vi "Receive Value Change Event.vi"(8 "error in (no error)":errorcluster, 10 "ValueChangeMsg":refnum<class "ValueChangeMsg.lvclass">, 11 "PauseResumeButtons In":refnum<class "PauseResumeButtons.lvclass">) -> (0 "error out":errorcluster, 3 "PauseResumeButtons Out":refnum<class "PauseResumeButtons.lvclass">)   [LabVIEW 2020, in "MVAExamples.lvlib" / "PauseResumeButtons.lvclass"]
doc: "<License>\nCopyright © 2017 Composed Systems, LLC | All rights reserved\nwww.composed.io\n\nAuthor: Ethan Stern <ethan.stern@composed.io>\n\nThis software is provided \"AS IS\" WITHOUT WARRANTIES, either express or implied, AND IS FOR EDUCATIONAL PURPOSES ONLY.\n</License>"
uses:
  PauseResumeButtons.lvclass
  modules/mva-viewable/Source/ActorEvents/IEventAggregator Messages/ValueChangeMsg/ValueChangeMsg.lvclass
  modules/mva-viewable/Source/ActorEvents/IEventAggregator Messages/ValueChangeMsg/ValueChangeMsg.lvclass/ValueChangeMsg.ctl
  PauseResumeButtons.lvclass/PauseResumeButtons.ctl
  modules/mva-viewable/Source/ActorEvents/IEventAggregator Messages/ValueChangeMsg/Accessors/Read Control Label.vi
  modules/mva-viewable/Source/IViewable/IViewable/IViewable.lvclass
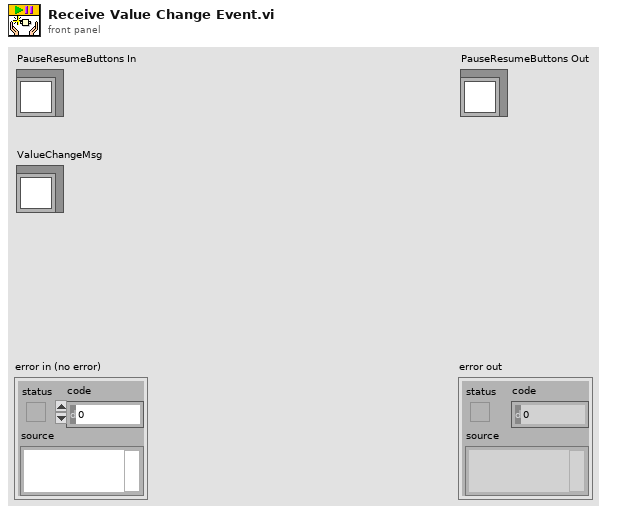
[diagram p1: front panel]
types:
  T1 = enum8{"Enabled", "Disabled", "Disabled and Grayed Out"}
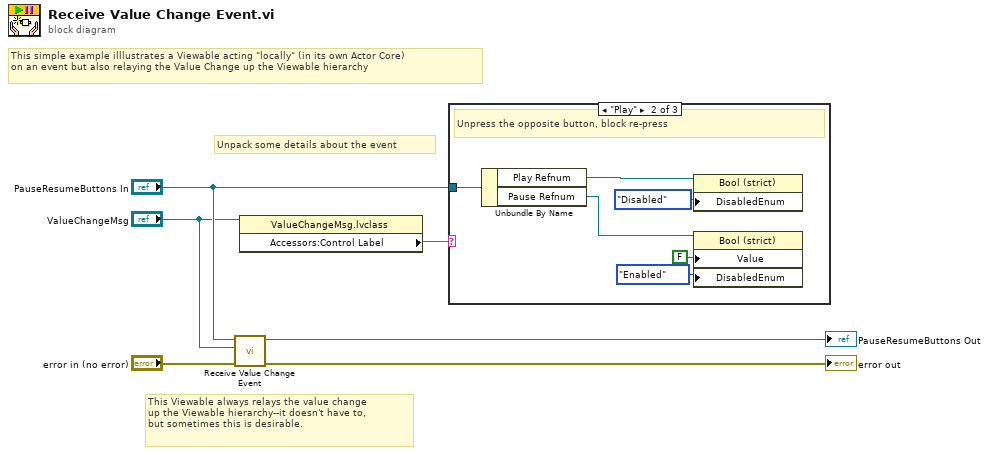
[diagram p0: block diagram]
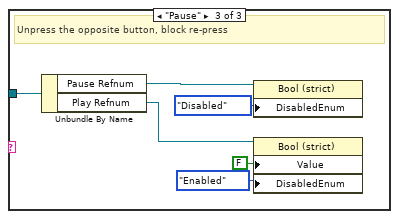
[diagram p3: hidden frame]
diagram:
  # "This simple example illlustrates a Viewable acting \"locally\" (in its own Actor Core)\non an event but also relaying the Value Change up the Viewable hierarchy"
  # "Unpack some details about the event"
  # "This Viewable always relays the value change\nup the Viewable hierarchy--it doesn't have to,\nbut sometimes this is desirable."
  n1 = call-parent "Receive Value Change Event.vi"("error in (no error)"="error in (no error)", "ValueChangeMsg"="ValueChangeMsg", "IViewable In"="PauseResumeButtons In") -> ("error out"=→"error out":errorcluster, "IViewable Out"=→"PauseResumeButtons Out":refnum<class "PauseResumeButtons.lvclass">)  [unwired: 7 in]
  n2 = property class="ValueChangeMsg.lvclass"(reference="ValueChangeMsg") -> ("Accessors:Control Label"=w1:string)  [unwired: 1 in, 2 out]
  n3 = case shown="\"Play\"" w1 {
    tunnel: "PauseResumeButtons In" -> [_ w12 w18]
    frame Default {
      # "Do nothing for unkown control"
    }
    frame "Play" {
      # "Unpress the opposite button, block re-press"
      n4 = Unbundle By Name(w12) -> ("Play Refnum"=w9:refnum<vi>, "Pause Refnum"=w11:refnum<vi>)
      n5 = property class="Bool (strict)"(reference=w9, "DisabledEnum"=T1."Disabled" ("Disabled")) -> ()  [unwired: 1 in, 2 out]
      n6 = property class="Bool (strict)"(reference=w11, "Value"=FALSE, "DisabledEnum"=T1."Enabled" ("Disabled")) -> ()  [unwired: 1 in, 2 out]
    }
    frame "Pause" {
      # "Unpress the opposite button, block re-press"
      n7 = Unbundle By Name(w18) -> ("Pause Refnum"=w15:refnum<vi>, "Play Refnum"=w17:refnum<vi>)
      n8 = property class="Bool (strict)"(reference=w15, "DisabledEnum"=T1."Disabled" ("Disabled")) -> ()  [unwired: 1 in, 2 out]
      n9 = property class="Bool (strict)"(reference=w17, "Value"=FALSE, "DisabledEnum"=T1."Enabled" ("Disabled")) -> ()  [unwired: 1 in, 2 out]
    }
  }
